vi "Lvi Write U16Data1D.vi"(7 "DataBuf":u16[](array[numeric])=array[4097 elements], 8 "error in (no error)":errorcluster, 9 "timeout":dbl, 10 "TaskRef":i32, 11 "NumSamples":u32) -> (0 "error out":errorcluster, 1 "function return":i32, 2 "TaskRef out":i32, 3 "NumQueued":u32)   [LabVIEW 2022 SP3, in "DtLvLink.lvlib"]
doc: "Calls directly into the entry points of the DLL of the Data Acq SDK to write a data point from the specified task as a one-dimensional array of unsigned, 16-bit integers."
uses:
  DtLvLink.lvlib
  <userlib>/LV-Link3/DtLvLink_64.dll
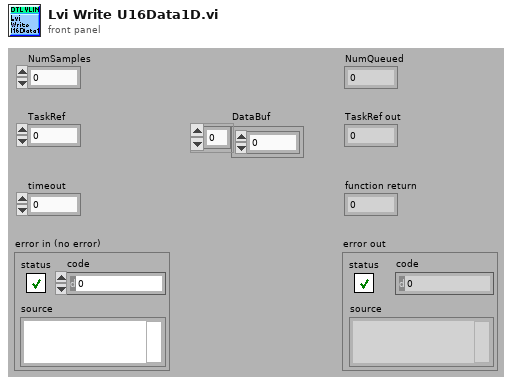
[diagram p1: front panel]
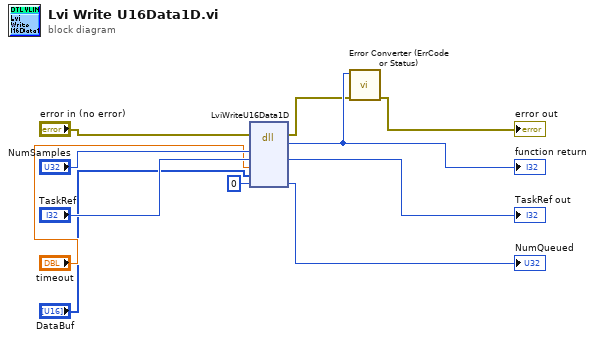
[diagram p0: block diagram]
diagram:
  n1 = dll-call lib="C:/Program Files/National Instruments/LabVIEW 2022/user.lib/LV-Link3/DtLvLink_64.*" fn="LviWriteU16Data1D"(error in="error in (no error)", "NumSamples"="NumSamples", "TaskRef"="TaskRef", "timeout"="timeout", "DataBuf"="DataBuf", "NumQueued"=u32 0) -> (error out=w2:errorcluster, "return type"=w11:i32, "TaskRef"=→"TaskRef out":i32, "NumQueued"=→"NumQueued":u32)  [unwired: 5 in, 1 out]
  "function return" <- w11
  n2 = call "Error Converter (ErrCode or Status).vi"("error in (no error)"=w2, "error code"=w11) -> ("error out"=→"error out":errorcluster)  [unwired: 9 in]
